vi "FreqWord.vi"(11 "Channel Frequency (MHz)":dbl format="%.6f") -> (1 "Actual Frequency (MHz)":dbl format="%.10f", 3 "Frequency Tuning Word":u32 format="%x")   [LabVIEW 2016]
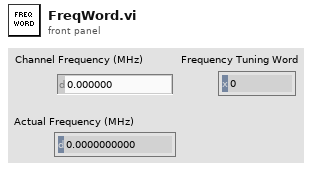
[diagram p1: front panel]
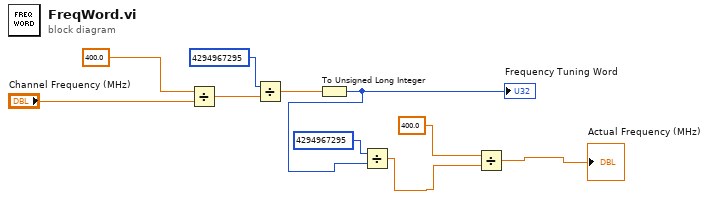
[diagram p0: block diagram]
diagram:
  n1 = Divide(x=400.0, y="Channel Frequency (MHz)") -> (x/y=w8:dbl)
  n2 = Divide(x=u32 4294967295, y=w8) -> (x/y=w5:dbl)
  n3 = To Unsigned Long Integer(number=w5) -> (unsigned 32bit integer=w3:u32)
  "Frequency Tuning Word" <- w3
  n4 = Divide(x=u32 4294967295, y=w3) -> (x/y=w2:dbl)
  n5 = Divide(x=400.0, y=w2) -> (x/y=→"Actual Frequency (MHz)":dbl)
